vi "generate 1 cycle.vi"(8 "error in (no error)":errorcluster caption="에러 입력(에러 없음)", 11 "Auto Tracking Wave 입력":refnum<class "Auto Track Wave.lvclass">) -> (0 "error out":errorcluster caption="에러 출력", 2 "waveform":waveform(dbl), 3 "Auto Tracking Wave 출력":refnum<class "Auto Track Wave.lvclass">)   [LabVIEW 2020, in "Auto Track Wave.lvclass"]
uses:
  Auto Track Wave.lvclass
  Waveform Gen/Waveform Gen.lvclass/Waveform Gen.ctl
  <vilib>/Waveform/WDTOps.llb/WDT Number of Waveform Samples DBL.vi
  Square Wave/Square Wave.lvclass
  Auto Track Wave.lvclass/Auto Track Wave.ctl
  Waveform Gen/Waveform Gen.lvclass
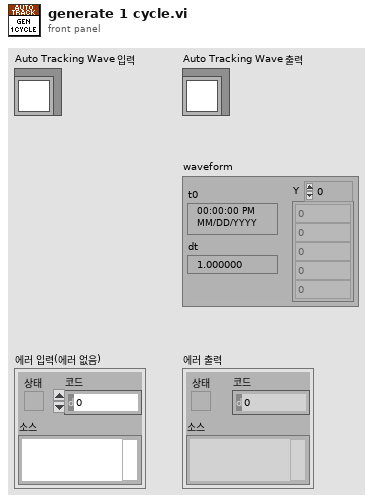
[diagram p1: front panel]
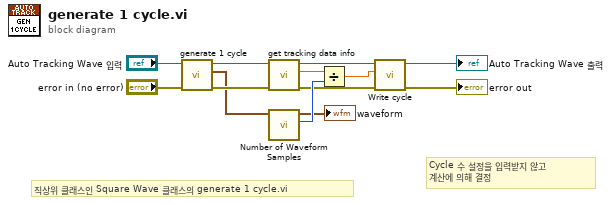
[diagram p0: block diagram]
diagram:
  # "Cycle 수 설정을 입력받지 않고\n계산에 의해 결정"
  # "직상위 클래스인 Square Wave 클래스의 generate 1 cycle.vi"
  n1 = call-parent "generate 1 cycle.vi"("error in (no error)"="error in (no error)", "Square Wave 입력"="Auto Tracking Wave 입력") -> ("error out"=w13:errorcluster, "waveform"=w9:waveform(dbl), "Square Wave 출력"=w10:refnum<class "Auto Track Wave.lvclass">)  [unwired: 7 in]
  n2 = call-dynamic "get tracking data info.vi"("error in (no error)"=w13, "Auto Tracking Wave 입력"=w10) -> ("error out"=w2:errorcluster, "wave length"=w7:dbl, "Auto Tracking Wave 출력"=w5:refnum<class "Auto Track Wave.lvclass">)  [unwired: 5 in, 2 out]
  n3 = call-poly <vilib>:"Number of Waveform Samples.vi"("waveform in"=w9) -> ("number of samples"=w8:i32, "waveform out"=→"waveform":waveform(dbl))  [unwired: 8 in, 1 out]
  n4 = Divide(x=w7, y=w8) -> (x/y=w1:dbl)
  n5 = call "Write cycle.vi"("error in (no error)"=w2, "cycle"=w1, "Waveform Obj 입력"=w5) -> ("error out"=→"error out":errorcluster, "Waveform Obj 출력"=→"Auto Tracking Wave 출력":refnum<class "Auto Track Wave.lvclass">)  [unwired: 7 in]
